vi "VIS-IR_SRingStartThread.vi"(6 "releasems":i16=2, 8 "error in (no error)":errorcluster, 9 "threadp":u32=31, 10 "ringdepth":u32, 11 "VIS-IR in":refnum<class "VIS-NIR.lvclass">) -> (0 "error out":errorcluster, 3 "VIS-IR out":refnum<class "VIS-NIR.lvclass">)   [LabVIEW 2015, in "VIS-NIR.lvclass"]
uses:
  VIS-NIR.lvclass
  Detector.lvclass/Detector.ctl
  Detector.lvclass
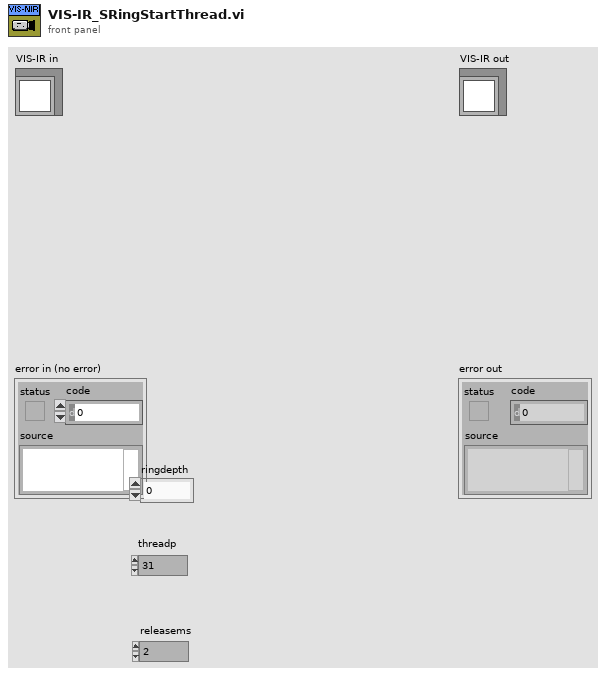
[diagram p1: front panel]
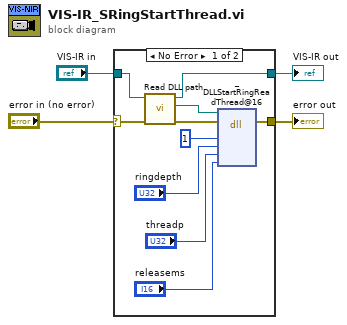
[diagram p0: block diagram]
diagram:
  n1 = case shown="No Error" "error in (no error)" {
    selector: "error in (no error)" -> [w13 w16]
    tunnel: [w8 w16] -> w3
    tunnel: [w5 w15] -> w1
    tunnel: "VIS-IR in" -> [w14 w15]
    frame No Error {
      n2 = call "Read DLL path.vi"("error in (no error)"=w13, "Detector in"=w14) -> ("error out"=w7:errorcluster, "DLL path"=w6:path, "Detector out"=w5:refnum<class "VIS-NIR.lvclass">)  [unwired: 7 in]
      n3 = dll-call lib="G:/SD/TRANCON/DLL/ESLSCDLL.dll" fn="_DLLStartRingReadThread@16" ("lwlscdll.dll:DLLStartRingReadThread")(path in=w6, error in=w7, "drv"=u32 1, "ringdepth"="ringdepth", "threadp"="threadp", "releasems"="releasems") -> (error out=w8:errorcluster)  [unwired: 6 in, 1 out]
    }
    frame Error {
    }
  }
  "error out" <- w3
  "VIS-IR out" <- w1
